vi "Configure Single Trigger.vi"(8 "error in (no error)":errorcluster, 9 "Enable Single Trigger (T: Enable)":bool=TRUE, 10 "Sample Count (1)":u32=1 min=1 max=1000, 11 "VISA resource name":refnum<visa-resource-name>) -> (0 "error out":errorcluster, 3 "VISA resource name out":refnum<visa-resource-name>)   [LabVIEW 2020, in "Library Instrument & Equipement.lvlib" / "Library Multimeter.lvlib" / "RIGOL DM3058.lvlib"]
doc: "Configures the Single Trigger parameter."
uses:
  RIGOL DM3058.lvlib
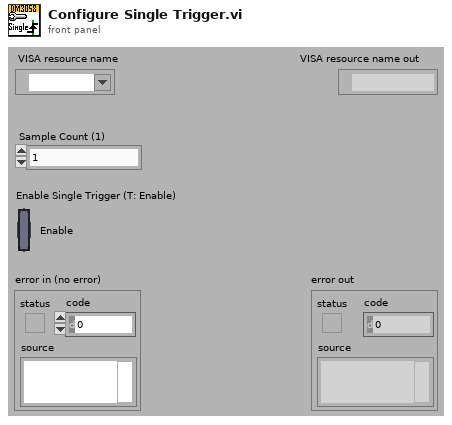
[diagram p1: front panel]
types:
  T1 = cluster{"DM Series Mode":u16, "Measurement Function":u16}
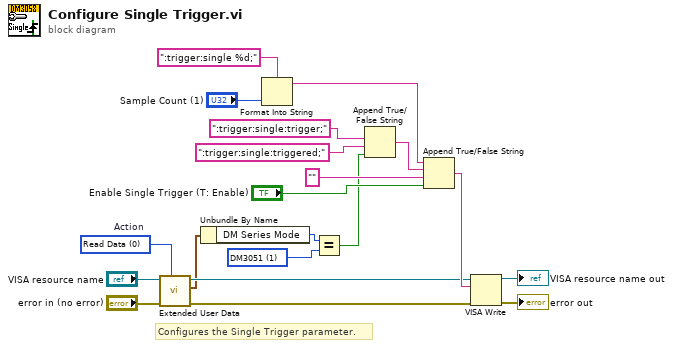
[diagram p0: block diagram]
diagram:
  w2 = u16 1 items=["DM3058", "DM3051", "DM3068", "DM3058E"] ("DM Series Mode")
  w8 = 0 items=["Read Data", "Write Data", "Clear Data", "Clear ALL Data"]  # Action
  # "Configures the Single Trigger parameter."
  n1 = call "Extended User Data.vi"("Action (1: Write Data)"=w8, "Error In (no error)"="error in (no error)", "VISA resource name in"="VISA resource name") -> ("Error Out"=w9:errorcluster, "User Data Out"=w1:T1, "VISA resource name out"=w10:refnum<visa-resource-name>)  [unwired: 1 in, 5 out]
  n2 = Unbundle By Name(w1) -> ("DM Series Mode"=w7:u16)
  n3 = Format Into String(format string=":trigger:single %d;" ("格式字符串"), "Sample Count (1)") -> (resulting string=w16:string)  [unwired: 2 in, 1 out]
  n4 = Equal?(x=w7, y=w2) -> (x = y?=w6:bool)
  n5 = Append True/False String(1:w6, 2:":trigger:single:triggered;" ("真字符串"), 3:":trigger:single:trigger;" ("true string")) -> (0:w5:string)  [unwired: 1 out]
  n6 = Append True/False String(1:"Enable Single Trigger (T: Enable)", 2:"" ("假字符串"), 3:w5, 4:w16) -> (0:w15:string)
  n7 = VISA Write(VISA resource name=w10, write buffer=w15, error in (no error)=w9) -> (VISA resource name out=→"VISA resource name out":refnum<visa-resource-name>, error out=→"error out":errorcluster)  [unwired: 1 out]
